vi "VisionTracking.vi"(11 "Image Refnum in":T1) -> (0 "Image Out":T1, 3 "Target Info":T2(array[cluster]))   [LabVIEW 2011]
uses:
  <vilib>/vision/Image Controls.llb/IMAQ Image.ctl
panel:
  in  "Annotate":bool=TRUE
  in  "Particle Count Limit":i32=10
  in  "Area Size Limit":i32=444
  in  "Score Limits":T3={"Rect Coverage"=76.0, "Aspect Ratio"=70.0, "X Edge Strength"=40.0, "Y Edge Strength"=60.0}
  in  "Camera Type":enum16{"206", "1011"}(ring)
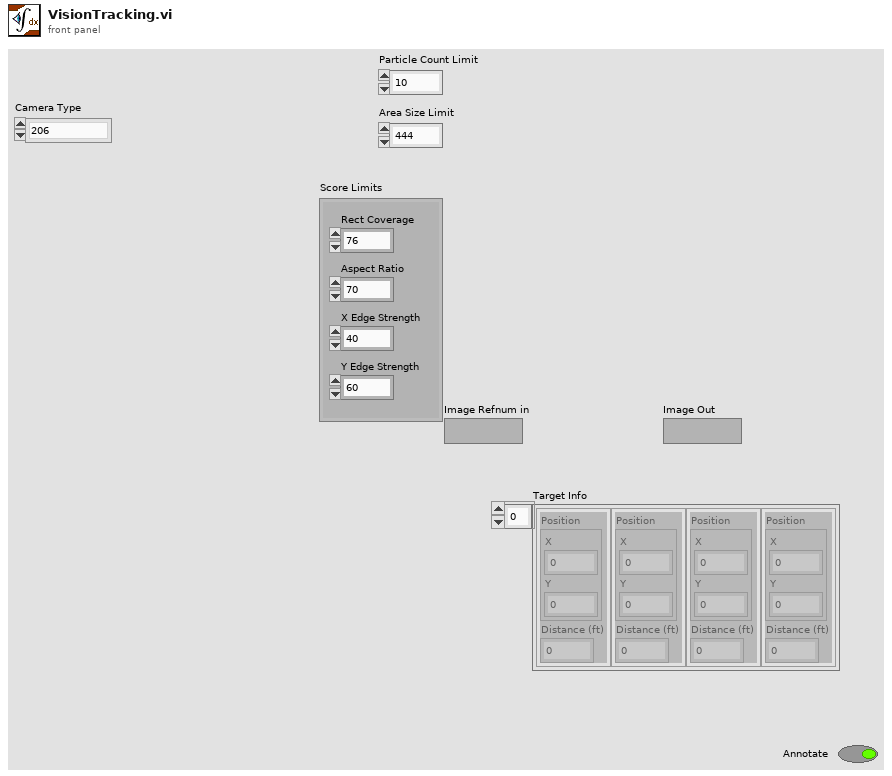
[diagram p1: front panel]
types:
  T1 = typedef "IMAQ Image.ctl" = refnum<image>
  T2 = cluster{"Position":cluster{"X":dbl, "Y":dbl}, "Distance (ft)":dbl}[]
  T3 = cluster{"Rect Coverage":dbl, "Aspect Ratio":dbl, "X Edge Strength":dbl, "Y Edge Strength":dbl}
  T4 = cluster{cluster{"Left":dbl, "Top":dbl, "Right":dbl, "Bottom":dbl}, dbl[]}[]
  T5 = cluster{"Left":dbl, "Top":dbl, "Right":dbl, "Bottom":dbl}
  T6 = cluster{"Target Center (-1 to 1)":cluster{"X":dbl, "Y":dbl}, "Distance (ft)":dbl}
  T7 = cluster{"Target Center (-1 to 1)":cluster{"X":dbl, "Y":dbl}, "Distance (ft)":dbl}[]
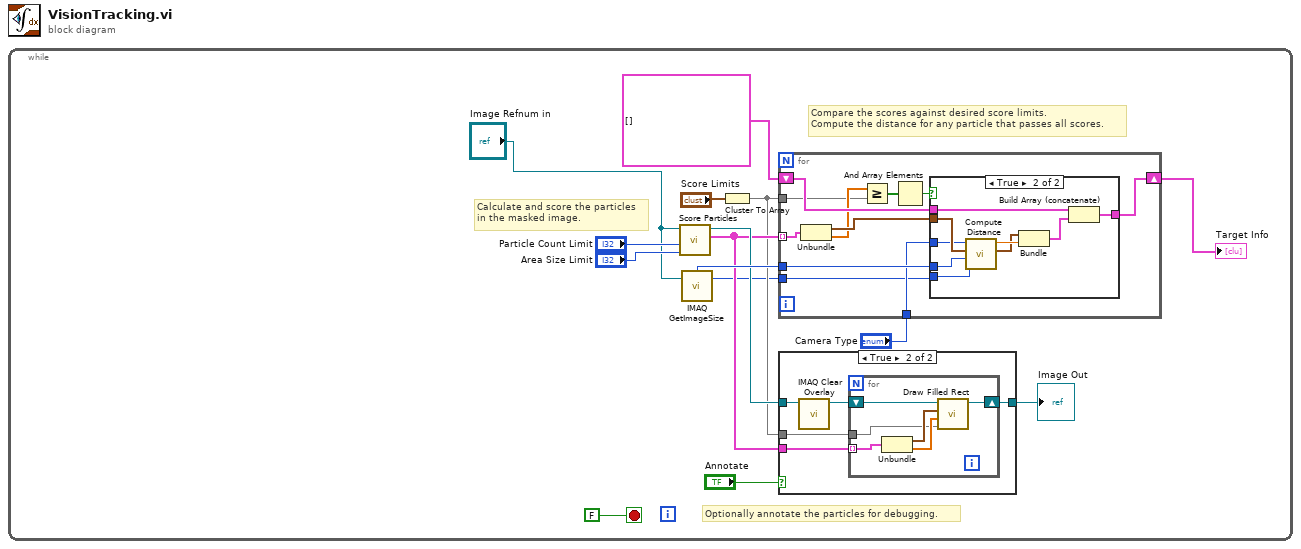
[diagram p0: block diagram]
diagram:
  n1 = while {
    stop <- FALSE stop-if-true
    # "Optionally annotate the particles for debugging."
    # "Compare the scores against desired score limits.\nCompute the distance for any particle that passes all scores."
    # "Calculate and score the particles\nin the masked image."
    n2 = call "Score Particles.vi"("Area Size Limit"="Area Size Limit", "Particle Count Limit"="Particle Count Limit", "Image Refnum in"="Image Refnum in") -> ("Scored Particle Info"=w10:T4, "Image Refnum out"=w13:T1)  [unwired: 7 in]
    n3 = call "IMAQ GetImageSize"("Image"="Image Refnum in") -> ("Y Resolution"=w4:i32, "X Resolution"=w14:i32)  [unwired: 3 in, 1 out]
    n4 = Cluster To Array(cluster="Score Limits") -> (array=w8:dbl[])
    n5 = for {
      shift-right: [w37] -> w3
      shift-left: T2 [] -> [w38]
      tunnel: w14 -> [w36]
      tunnel: w10 -> [w34] mode=indexing
      tunnel: w8 -> [w29]
      tunnel: "Camera Type" -> [w33]
      tunnel: w4 -> [w28]
      n6 = Unbundle(w34) -> (w35:T5, w30:dbl[])
      n7 = Greater Or Equal?(x=w30, y=w29) -> (x >= y?=w32:bool[])
      n8 = And Array Elements(Boolean array=w32) -> (logical AND=w31:bool)
      n9 = case shown="True" w31 {
        tunnel: w38 -> [w39 w48]
        tunnel: [w39 w47] -> w37
        tunnel: w35 -> [_ w43]
        tunnel: w36 -> [_ w45]
        tunnel: w33 -> [_ w42]
        tunnel: w28 -> [_ w40]
        frame False {
        }
        frame True {
          n10 = call "Compute Distance.vi"("Y Image Resolution"=w40, "X Image Resolution"=w45, "Bounding Box"=w43, "Camera Type"=w42) -> ("Target Center (-1 to 1)"=w41:cluster{"X":dbl, "Y":dbl}, "Distance (ft)"=w44:dbl)  [unwired: 6 in]
          n11 = Bundle("Target Center (-1 to 1)"=w41, "Distance (ft)"=w44) -> (w46:T6)  [unwired: 1 in]
          n12 = Build Array (concatenate)(w48, w46) -> (w47:T7)
        }
      }
    }
    "Target Info" <- w3
    n13 = case shown="True" "Annotate" {
      tunnel: w13 -> [w16 w21]
      tunnel: [w16 w20] -> w2
      tunnel: w10 -> [_ w18]
      tunnel: w8 -> [_ w17]
      frame False {
      }
      frame True {
        n14 = call "IMAQ Clear Overlay"("Image"=w21) -> ("Image Out"=w19:T1)  [unwired: 2 in, 8 out]
        n15 = for {
          shift-right: [w26] -> w20
          shift-left: w19 -> [w27]
          tunnel: w18 -> [w23] mode=indexing
          tunnel: w17 -> [w22]
          n16 = Unbundle(w23) -> (w24:T5, w25:dbl[])
          n17 = call "Draw Filled Rect.vi"("Limits"=w22, "Scores"=w25, "Bounding Box"=w24, "image in"=w27) -> ("image out"=w26:T1)  [unwired: 7 in]
        }
      }
    }
    "Image Out" <- w2
  }
